vi "Send Configure Sample Clock [SC].vi"(7 "Message Priority (Normal)":T1=enum."Normal", 8 "error in (no error)":errorcluster, 10 "Sample Clock Source (Internal)":i32(ring) items=["Internal", "External"], 11 "Message Enqueuer":refnum<class "Message Enqueuer.lvclass">) -> (0 "error out":errorcluster, 3 "Message Enqueuer out":refnum<class "Message Enqueuer.lvclass">)   [LabVIEW 2015, in "CS++Fgen.lvlib" / "Configure Sample Clock [SC] Msg.lvclass"]
doc: "Sends the <B>CS++Fgen.lvlib:Configure Sample Clock [SC] Msg.lvclass</B> message.\n\n<B>CS++Fgen.lvlib:CS++Fgen.lvclass:Configure Sample Clock [SC].vi</B> Description:\n\nThis VI configures the sample clock source for the function generator. \n\nNote:\n\n(1) This VI is part of the IviFgenSampleClock [SC] extension group."
uses:
  Configure Sample Clock [SC] Msg.lvclass
  <vilib>/ActorFramework/Message Enqueuer/Message Enqueuer.lvclass
  <vilib>/ActorFramework/Message Enqueuer/Message Priority.ctl
  Configure Sample Clock [SC] Msg.lvclass/Configure Sample Clock [SC] Msg.ctl
  <vilib>/ActorFramework/Message Enqueuer/Message Enqueuer.lvclass/Message Enqueuer.ctl
  <vilib>/ActorFramework/Message Priority Queue/Priority Enqueue.vi
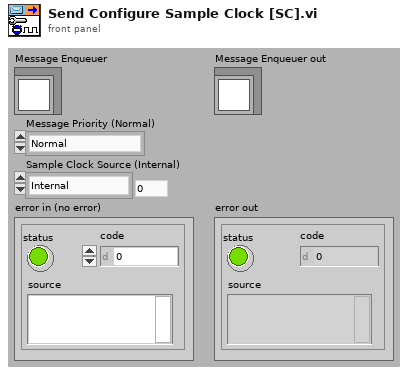
[diagram p1: front panel]
types:
  T1 = typedef "Actor Framework.lvlib/Message Enqueuer.lvclass/Message Priority.ctl" = enum16{"Low", "Normal", "High"}
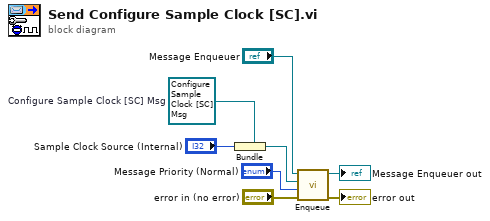
[diagram p0: block diagram]
diagram:
  w2 = refnum<class "Configure Sample Clock [SC] Msg.lvclass"> refnum  # Configure Sample Clock [SC] Msg
  n1 = Bundle(cluster=w2, "Sample Clock Source (Internal)") -> (w5:refnum<class "Configure Sample Clock [SC] Msg.lvclass">)
  n2 = call <vilib>:"Enqueue.vi"("error in (no error)"="error in (no error)", "Message Priority (Normal)"="Message Priority (Normal)", "Message"=w5, "Message Enqueuer in"="Message Enqueuer") -> ("error out"=→"error out":errorcluster, "Message Enqueuer out"=→"Message Enqueuer out":refnum<class "Message Enqueuer.lvclass">)  [unwired: 6 in]
